vi "Convert Content into Name.vi"(8 "Error In":errorcluster, 11 "Content":string) -> (0 "Error Out":errorcluster, 3 "Name":string[](array[string]))   [LabVIEW 2017, in "Mustache.lvlib" / "Parser.lvclass"]
uses:
  Parser.lvclass
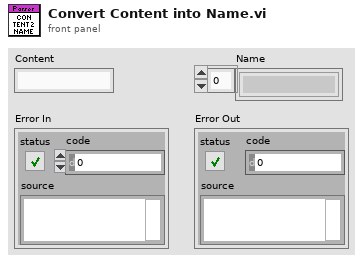
[diagram p1: front panel]
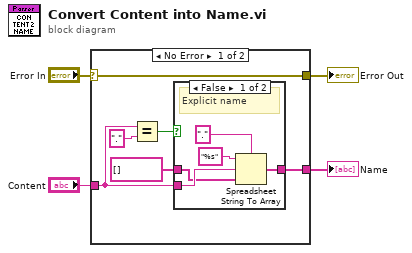
[diagram p0: block diagram]
diagram:
  n1 = case shown="No Error" "Error In" {
    selector: "Error In" -> [w5 w17]
    tunnel: [w10 _] -> w4
    tunnel: "Content" -> [w9 _]
    tunnel: [w5 w17] -> w1
    frame No Error {
      n2 = Equal?(x=w9, y=".") -> (x = y?=w7:bool)
      n3 = case shown="False" w7 {
        tunnel: w9 -> [w13 _]
        tunnel: [w12 w16] -> w10
        tunnel: string[] [] -> [w11 w16]
        frame False {
          # "Explicit name"
          n4 = Spreadsheet String To Array(delimiter (Tab)=".", format string="%s", spreadsheet string=w13, array type (2D Dbl)=w11) -> (array=w12:string[])
        }
        frame True {
          # "Implicit name"
        }
      }
    }
    frame Error {
    }
  }
  "Name" <- w4
  "Error Out" <- w1
